vi "Voltage_Measurement_from_3457A.vi"(8 "error in":errorcluster) -> (0 "error out":errorcluster, 2 "mean":dbl format="%0.6f")   [LabVIEW 2020]
uses:
  <vilib>/Analysis/baseanly.llb/Mean (DBL).vi
  <vilib>/Analysis/NI_AALBase.lvlib
panel:
  out "Sample Array":dbl[](array[numeric])
  in  "Voltage Set 2":dbl format="%.6g"
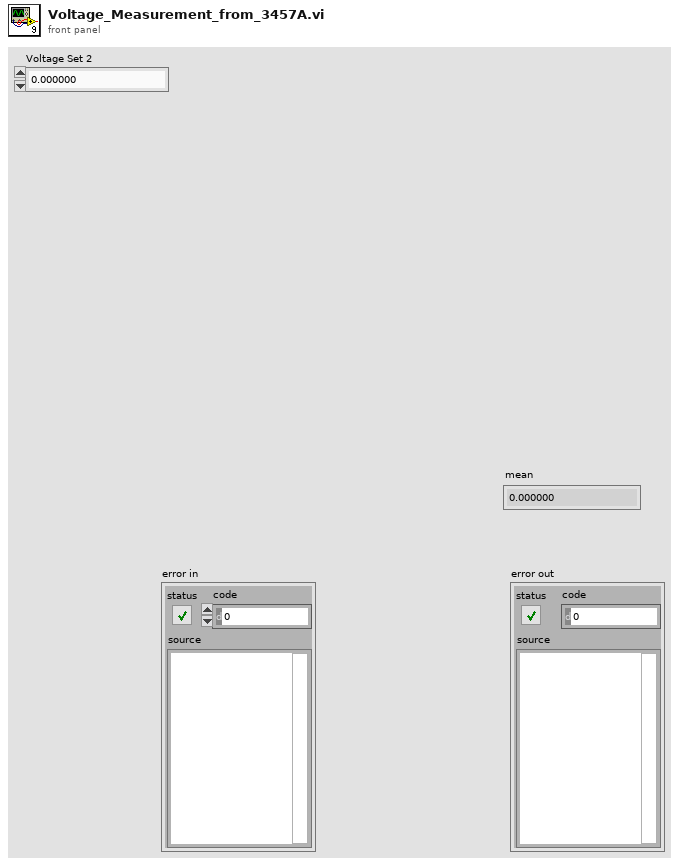
[diagram p1: front panel]
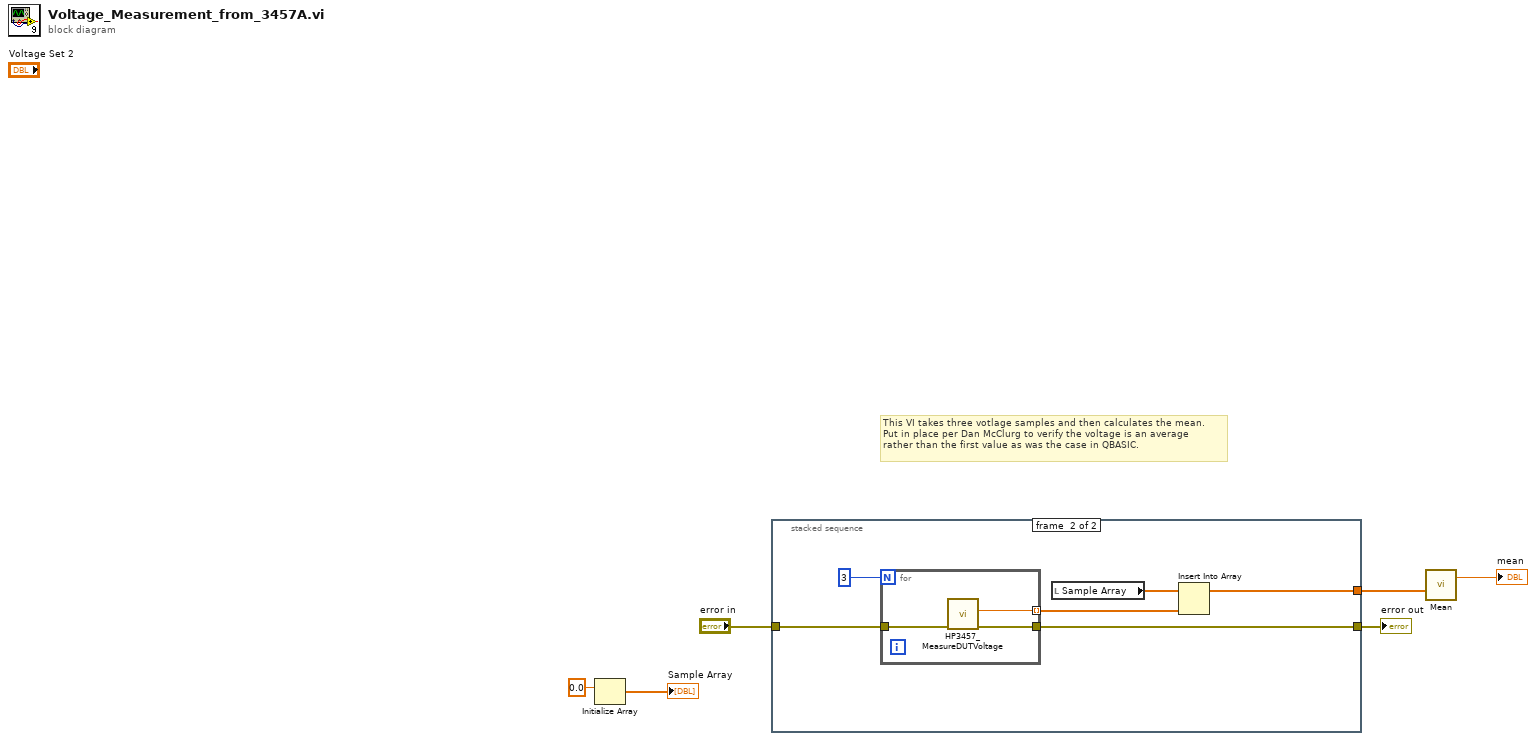
[diagram p0: block diagram]
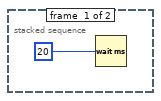
[diagram p2: hidden frame]
diagram:
  # "This VI takes three votlage samples and then calculates the mean.\nPut in place per Dan McClurg to verify the voltage is an average\nrather than the first value as was the case in QBASIC."
  n1 = Initialize Array(0.0 ("element")) -> (→"Sample Array":dbl[])  [unwired: 1 in]
  n2 = stacked-sequence {
    tunnel: "error in" -> [_ w11]
    tunnel: [_ w9] -> w3
    tunnel: [_ w8] -> w2
    frame #0 {
      n3 = Wait (ms)(milliseconds to wait=u32 20) -> ()  [unwired: 1 out]
    }
    frame #1 {
      n4 = for {
        N: 3 -> [_]
        tunnel: [w16] -> w12 mode=indexing
        tunnel: w11 -> [w15]
        tunnel: [w14] -> w9
        n5 = call "HP3457_MeasureDUTVoltage.vi"("error in"=w15) -> ("error out"=w14:errorcluster, "DUTVoltage"=w16:dbl)  [unwired: 8 in]
      }
      n6 = local read "Sample Array"() -> (w10:dbl[])
      n7 = Insert Into Array(array=w10, new element=w12) -> (w8:dbl[])  [unwired: 1 in]
    }
  }
  "error out" <- w3
  n8 = call-poly <vilib>:"Mean.vi"("X"=w2) -> ("mean"=→"mean":dbl)  [unwired: 1 out]
